vi "Arduino Photocell.vi"() -> ()   [LabVIEW 2014, in "LabVIEW Interface for Arduino.lvlib"]
doc: "An example that uses the Arduino to read the value of a photocell."
uses:
  <vilib>/LabVIEW Interface for Arduino/LabVIEW Interface for Arduino.lvlib
  <vilib>/LabVIEW Interface for Arduino/Type Defs/Analog Pin.ctl
panel:
  in  "VISA resource":refnum<visa-resource-name>
  in  "Stop":bool
  out "Light Intensity (0 - 100)":dbl(knob) scale=0.0..100.0
  in  "Photo Cell Pin (AI 0-5)":T1=enum."Anlog In 1"
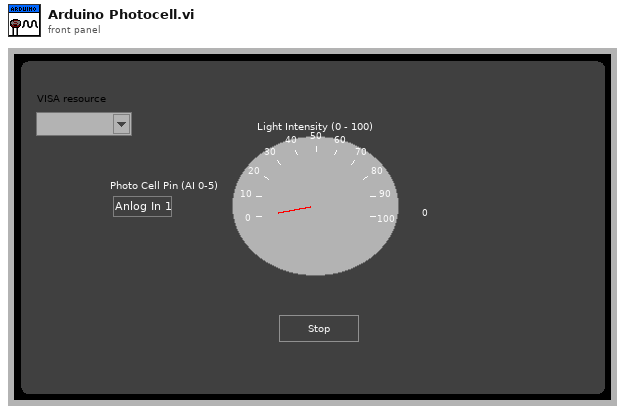
[diagram p1: front panel]
types:
  T1 = typedef "LabVIEW Interface for Arduino.lvlib/Analog Pin.ctl" = enum8{"Anlog In 0", "Anlog In 1", "Anlog In 2", "Anlog In 3", "Anlog In 4", "Anlog In 5"}
  T2 = typedef "LabVIEW Interface for Arduino.lvlib/Arduino Resource.ctl" = cluster{"VISA resource":refnum<visa-resource-name>, "Board Type":T3, "Connection Type":enum8{"USB / Serial"}, "Bytes Per Packet (15)":u8}
  T3 = typedef "LabVIEW Interface for Arduino.lvlib/Board Type.ctl" = enum16{"Uno", "Dimuelanove w/Atmega 328", "Mega 2560"}
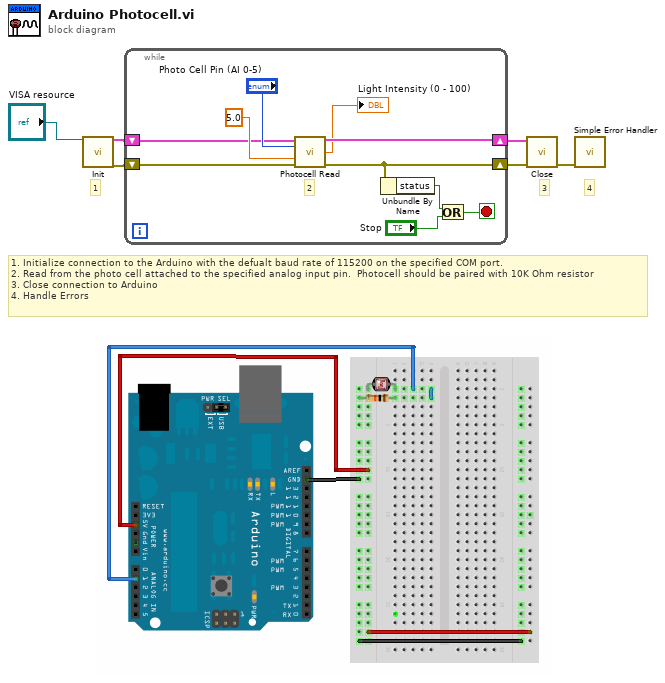
[diagram p0: block diagram]
diagram:
  # "1. Initialize connection to the Arduino with the defualt baud rate of 115200 on the specified COM port.\n2. Read from the photo cell attached to the specified analog input pin.  Photocell should be paired with 10K Ohm resistor\n3. Close connection to Arduino\n4. Handle Errors"
  # "4"
  # "3"
  # "1"
  n1 = call <vilib>:"Init.vi"("VISA resource"="VISA resource") -> ("Arduino Resource"=w5:T2, "error out"=w4:errorcluster)  [unwired: 17 in]
  n2 = while {
    shift-right: [w12] -> w6
    shift-left: w4 -> [w16]
    shift-right: [w15] -> w2
    shift-left: w5 -> [w8]
    stop <- w9 stop-if-true
    # "2"
    n3 = call <vilib>:"Photocell Read.vi"("Arduino Resource"=w8, "Photo Cell Pin (0)"="Photo Cell Pin (AI 0-5)", "Vcc (5)"=5.0 ("Vcc"), "error in"=w16) -> ("Arduino Resource"=w15:T2, "Light Intensity (0 - 100)"=→"Light Intensity (0 - 100)":dbl, "error out"=w12:errorcluster)  [unwired: 9 in]
    n4 = Unbundle By Name(w12) -> ("status"=w11:bool)
    n5 = Or(x=w11, y="Stop") -> (x .or. y?=w9:bool)
  }
  n6 = call <vilib>:"Close.vi"("Arduino Resource"=w2, "error in"=w6) -> ("error out"=w3:errorcluster)  [unwired: 13 in]
  n7 = call <vilib>:"Simple Error Handler.vi"("error in (no error)"=w3) -> ()  [unwired: 4 in, 5 out]
